vi "Kelompok 3_For Loop.vi"() -> ()   [LabVIEW 2020]
uses:
  <vilib>/numeric/Random Number (Range) I64.vi
  <vilib>/numeric/sub_Random U32.vi
panel:
  out "Output 2":i64
  out "Array":i64[](array[numeric])
  out "output":i64
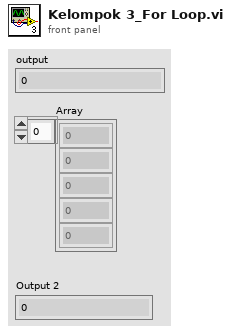
[diagram p1: front panel]
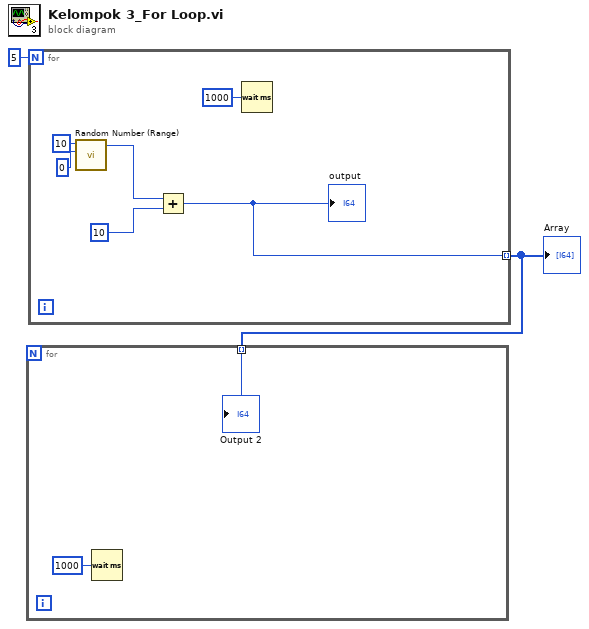
[diagram p0: block diagram]
diagram:
  n1 = for {
    N: 5 -> [_]
    tunnel: [w3] -> w1 mode=indexing
    n2 = call-poly <vilib>:"Random Number (Range).vi"("lower bound (-100)"=i64 0, "upper bound (100)"=i64 10) -> ("number"=w6:i64)  [unwired: 9 in]
    n3 = Add(x=w6, y=i64 10) -> (x+y=w3:i64)
    "output" <- w3
    n4 = Wait (ms)(milliseconds to wait=u32 1000) -> ()  [unwired: 1 out]
  }
  "Array" <- w1
  n5 = for {
    tunnel: w1 -> [w9] mode=indexing
    n6 = Wait (ms)(milliseconds to wait=u32 1000) -> ()  [unwired: 1 out]
    "Output 2" <- w9
  }
